vi "Get part number info block from text file.vi"(8 "error in (no error)":errorcluster, 10 "StylePartNum":string, 11 "file (use dialog)":path) -> (0 "error out":errorcluster, 2 "Found part number info":bool, 3 "Info block":string)   [LabVIEW 2024]
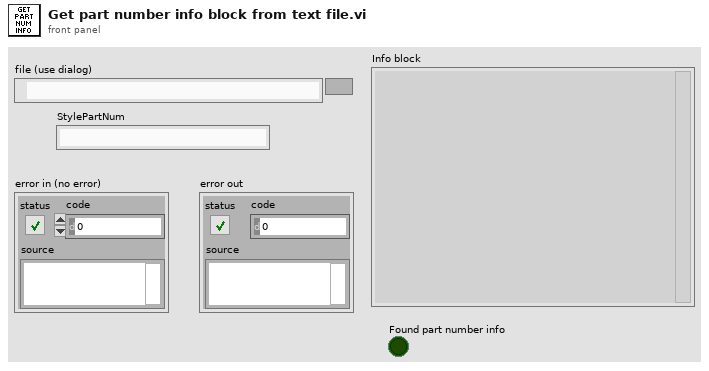
[diagram p1: front panel]
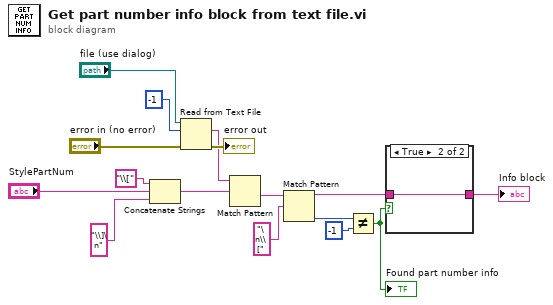
[diagram p0: block diagram]
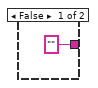
[diagram p2: hidden frame]
diagram:
  n1 = Concatenate Strings("\\[" ("string"), "StylePartNum", "\\]\n" ("string")) -> (w12:string)
  n2 = Read from Text File(file (use dialog)="file (use dialog)", count=-1, error in="error in (no error)") -> (text=w9:string, error out=→"error out":errorcluster)  [unwired: 1 in, 2 out]
  n3 = Match Pattern(string=w9, regular expression=w12) -> (after substring=w13:string)  [unwired: 1 in, 3 out]
  n4 = Match Pattern(string=w13, regular expression="\n\\[") -> (before substring=w5:string, offset past match=w4:i32)  [unwired: 1 in, 2 out]
  n5 = Not Equal?(x=w4, y=-1) -> (x != y?=w2:bool)
  "Found part number info" <- w2
  n6 = case shown="True" w2 {
    tunnel: w5 -> [_ w18]
    tunnel: ["" w18] -> w1
    frame False {
    }
    frame True {
    }
  }
  "Info block" <- w1
